vi "Get Current View.vi"(5 "Team Index":i32, 7 "View":i32[](array[numeric]) caption="View (Team Index, -1: empty)", 9 "Column":i32, 10 "Row":i32, 11 "Move Array":i32[][](array[numeric])) -> (1 "New View Out":i32[](array[numeric]), 2 "Directions Out":T1[](array[typedef])=[enum."NW", enum."N", enum."NE", enum."E", enum."SE", enum."S", enum."S", enum."SW", enum."W"], 3 "Move Array":i32[][](array[numeric]))   [LabVIEW 2017, in "AntFarm_MB.lvclass"]
uses:
  AntFarm_MB.lvclass
  Type Defs/Direction Enum.ctl
  Type Defs/SB Type Defs.lvlib
panel:
  # "ww"
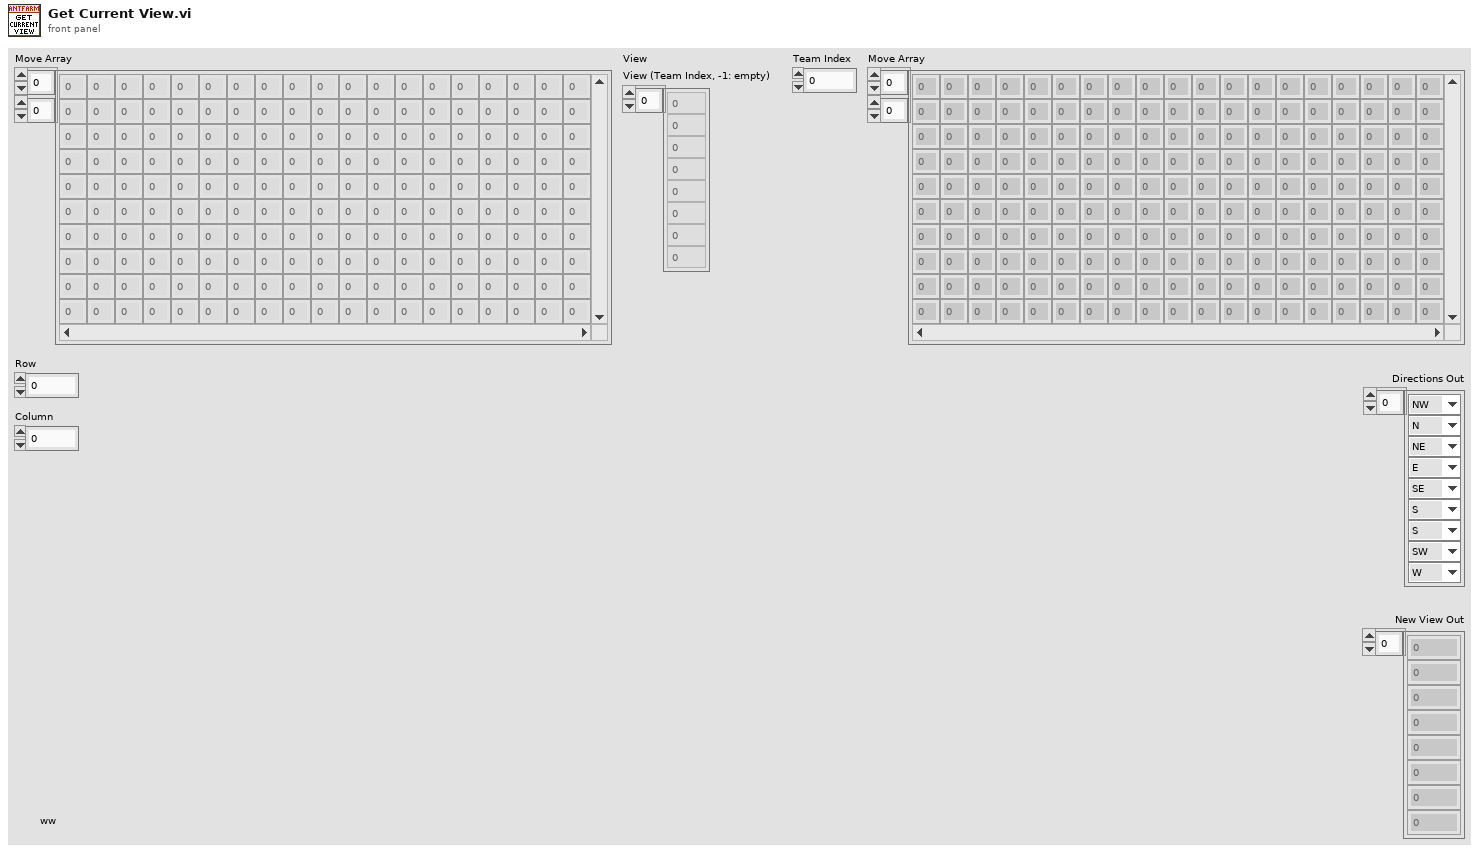
[diagram p1: front panel]
types:
  T1 = typedef "SB Type Defs.lvlib/Direction Enum.ctl" = enum16{"NW", "N", "NE", "E", "SE", "S", "SW", "W"}
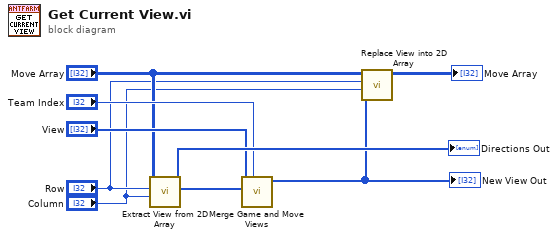
[diagram p0: block diagram]
diagram:
  n1 = call "Extract View from 2D Array.vi"("Column"="Column", "Row"="Row", "Board Array"="Move Array") -> ("View Out"=w7:i32[], "Directions Out"=→"Directions Out":T1[])  [unwired: 7 in]
  n2 = call "Merge Game and Move Views.vi"("Team Index"="Team Index", "Move View Out"=w7, "System View Out"="View") -> ("New View Out"=w1:i32[])  [unwired: 8 in]
  "New View Out" <- w1
  n3 = call "Replace View into 2D Array.vi"("View"=w1, "Column"="Column", "Row"="Row", "Board Array"="Move Array") -> ("Board Array Out"=→"Move Array":i32[][])  [unwired: 7 in]
